vi "Acquire Block.vi"(8 "error in":errorcluster, 10 "start sample":dbl, 11 "generator settings":T1={"Amplitude"=1.0, "Frequency"=10.0, "Sample Rate"=1000.0, "Noise Level"=0.0, "Signal Type"=enum."Sine", "Block Size"=100, "Update Interval ms"=100}) -> (0 "error out":errorcluster, 2 "next start sample":dbl, 3 "waveform":cluster{"x_data":dbl[], "y_data":dbl[]})   [LabVIEW 2026, in "Signal Generator.lvlib"]
doc: "Acquisition stage. Produces the next block of synthetic waveform data as an XY pair (time in seconds, signal value) by calling the signal generation engine, and returns the absolute sample index at which the following block must start. No hardware is accessed."
uses:
  Signal Generator.lvlib
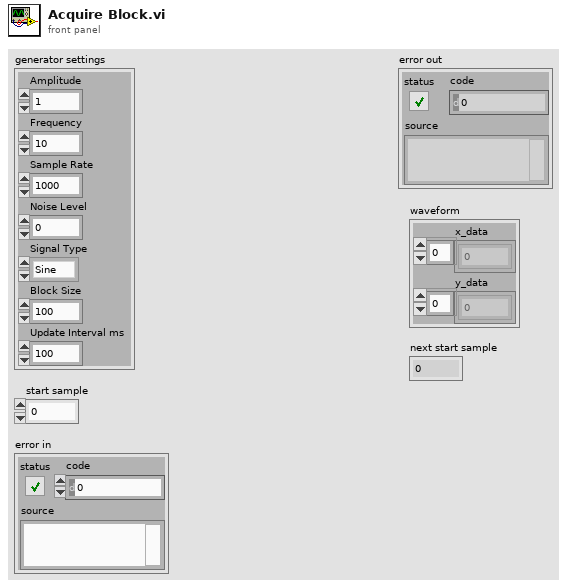
[diagram p1: front panel]
types:
  T1 = cluster{"Amplitude":dbl, "Frequency":dbl, "Sample Rate":dbl, "Noise Level":dbl, "Signal Type":enum32{"Sine", "Square", "Chirp"}, "Block Size":i32, "Update Interval ms":i32}
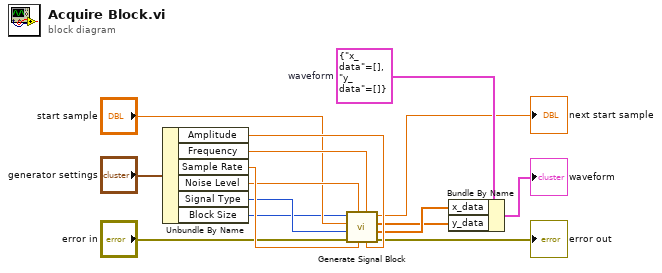
[diagram p0: block diagram]
diagram:
  w4 = cluster{"x_data":dbl[], "y_data":dbl[]} {"x_data"=[], "y_data"=[]}  # waveform
  n1 = Unbundle By Name("generator settings") -> ("Amplitude"=w14:dbl, "Frequency"=w13:dbl, "Sample Rate"=w12:dbl, "Noise Level"=w11:dbl, "Signal Type"=w9:enum32{"Sine", "Square", "Chirp"}, "Block Size"=w7:i32)
  n2 = call "Generate Signal Block.vi"("amplitude"=w14, "frequency"=w13, "sample rate"=w12, "noise level"=w11, "error in"="error in", "signal type"=w9, "start sample"="start sample", "samples"=w7) -> ("error out"=→"error out":errorcluster, "time"=w6:dbl[], "signal"=w5:dbl[], "next start sample"=→"next start sample":dbl)
  n3 = Bundle By Name(cluster=w4, "x_data"=w6, "y_data"=w5) -> (→"waveform":cluster{"x_data":dbl[], "y_data":dbl[]})
